vi "New Alias UI.vi"(10 "Picture":picture, 11 "Current Alias":string) -> (2 "Cancelled":bool, 3 "Alias":string)   [LabVIEW 2020, in "PicoG-App.lvlib" / "DeviceDetailPanel.lvclass"]
uses:
  DeviceDetailPanel.lvclass
  <vilib>/event_ctls.llb/eventvkey.ctl
panel:
  in  "Cancel":bool
  in  "OK":bool
  # "Please enter the new Alias to assign to this device:"
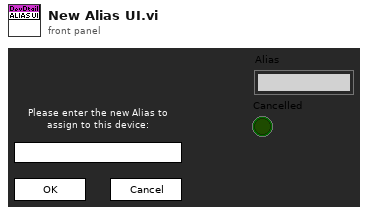
[diagram p1: front panel]
types:
  T1 = typedef "eventvkey.ctl" = enum16{"ASCII", "Enter", "Return", "Shift", "Ctrl", "Alt", "Cmd", "Opt", "Caps", "NumLock", "Clear", "Break", "Up", "Down", "Left", "Right", "Insert", "Delete", "Home", "End", "PageUp", "PageDown", "Escape", "Help", "Pause", "ScrollLock", "F1", "F2", "F3", "F4", "F5", "F6", "F7", "F8", "F9", "F10", "F11", "F12", "F13", "F14", "F15", "F16", "F17", "F18", "F19", "F20", "F21", "F22", "F23", "F24", "Play", "VolumeUp", "VolumeDown", "Mute", "Two Byte Char"}
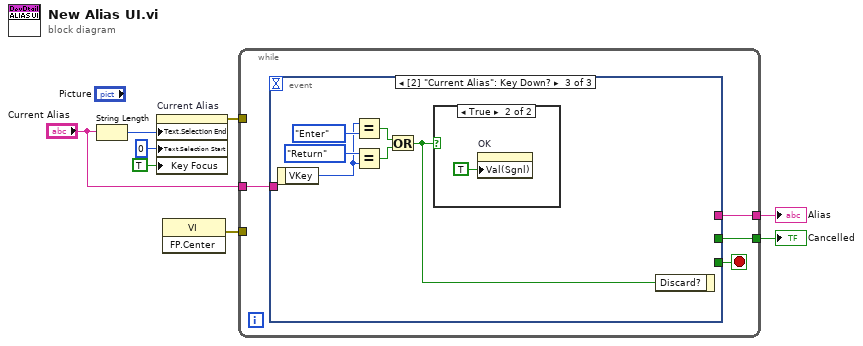
[diagram p0: block diagram]
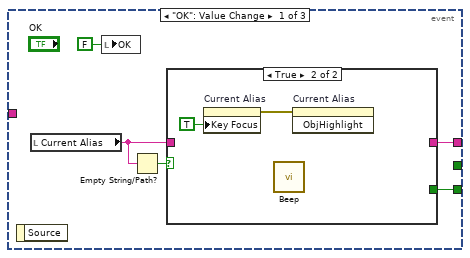
[diagram p2: hidden frame]
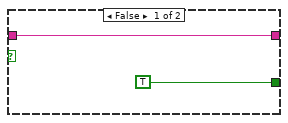
[diagram p3: hidden frame]
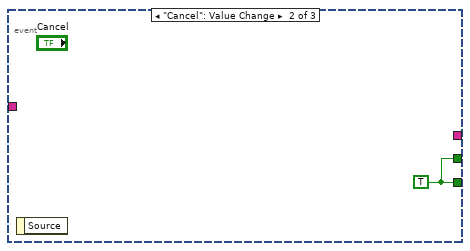
[diagram p4: hidden frame]
diagram:
  n1 = String Length(string="Current Alias") -> (length=w6:i32)
  n2 = property on="Current Alias" class="Str"("Text.Selection End"=w6, "Text.Selection Start"=u32 0 ("Text.Selection:Start"), "Key Focus"=TRUE) -> (error out=w4:errorcluster)  [unwired: 2 in, 1 out]
  n3 = invoke class="VI" method="FP.Center"() -> (error out=w8:errorcluster)  [unwired: 3 in, 2 out]
  n4 = while {
    tunnel: w8 -> [_]
    tunnel: w4 -> [_]
    tunnel: "Current Alias" -> [w12]
    tunnel: [w11] -> w2
    tunnel: [w9] -> w1
    stop <- w10 stop-if-true
    n5 = event shown="[2] \"Current Alias\": Key Down?" {
      selector: _ -> [_ _ _]
      dyn-events: _ -> [_ _ _]
      timeout: _ -> [_ _ _]
      tunnel: w12 -> [_ _ _]
      tunnel: [w14 _ _] -> w11
      tunnel: [w13 w22 _] -> w10
      tunnel: [_ w22 _] -> w9
      event "OK": Value Change {
        n6 = event-data() -> ()  [unwired: 1 in, 1 out]
        n7 = local read "Current Alias"() -> (w15:string)
        n8 = local write "OK"(FALSE ("OK")) -> ()
        n9 = Empty String/Path?(string/path=w15) -> (empty?=w16:bool)
        n10 = case shown="True" w16 {
          tunnel: w15 -> [w19 _]
          tunnel: [w19 _] -> w14
          tunnel: [TRUE _] -> w13
          frame False {
          }
          frame True {
            n11 = property on="Current Alias" class="Str"("Key Focus"=TRUE) -> (error out=w20:errorcluster)  [unwired: 2 in, 1 out]
            n12 = call <vilib>:"Beep.vi"() -> ()  [unwired: 12 in]
            n13 = invoke on="Current Alias" class="Str" method="ObjHighlight"(error in=w20) -> ()  [unwired: 2 in, 3 out]
          }
        }
      }
      event "Cancel": Value Change {
        w22 = TRUE
        n14 = event-data() -> ()  [unwired: 1 in, 1 out]
      }
      event "Current Alias": Key Down? {
        n15 = event-data() -> ("VKey"=w26:T1)  [unwired: 1 in]
        n16 = Equal?(x=w26, y=eventvkey."Enter" ("VKey")) -> (x = y?=w25:bool)
        n17 = Equal?(x=eventvkey."Return" ("VKey"), y=w26) -> (x = y?=w24:bool)
        n18 = Or(x=w25, y=w24) -> (x .or. y?=w23:bool)
        n19 = case shown="True" w23 {
          frame False {
          }
          frame True {
            n20 = property on="OK" class="Bool (strict)"("Val(Sgnl)"=TRUE ("Value (Signaling)")) -> ()  [unwired: 2 in, 2 out]
          }
        }
        n21 = event-data("Discard?"=w23) -> ()  [unwired: 1 in, 1 out]
      }
    }
  }
  "Alias" <- w2
  "Cancelled" <- w1
